vi "IRCalibration.vi"() -> ()   [LabVIEW 2017]
panel:
  out "interpolation value":dbl
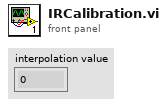
[diagram p1: front panel]
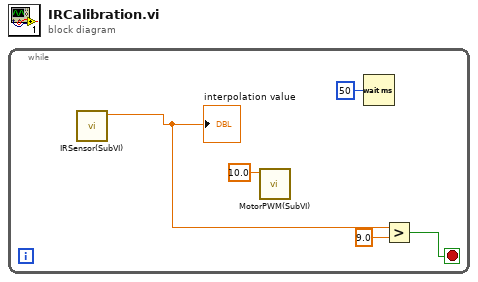
[diagram p0: block diagram]
diagram:
  n1 = while {
    stop <- w2 stop-if-true
    n2 = call "IRSensor(SubVI).vi"() -> ("interpolation value"=w3:dbl)  [unwired: 11 in]
    "interpolation value" <- w3
    n3 = call "MotorPWM(SubVI).vi"("Duty Cycle (-100 to + 100)"=10.0) -> ()  [unwired: 11 in]
    n4 = Wait (ms)(milliseconds to wait=u32 50) -> ()  [unwired: 1 out]
    n5 = Greater?(x=w3, y=9.0) -> (0:w2:bool)
  }
